vi "Load Named Colors.vi"() -> ()   [LabVIEW 2015, in "ColorSelector.lvclass"]
doc: "This VI is a scripting VI that edits the <b>Named Colors Enum</b> and creates the named colors lookup table from the list in the <b>Named Colors List Text File</b>.\n<b> </b> <b> </b>\n©2017 Q Software Innovations, LLC (QSI)\nwritten by Quentin Alldredge\nproduced in LabVIEW 2015\n\nsupport@qsoftwareinnovations.com\nwww.qsoftwareinnovations.com\n\nAll rights reserved.\n\nRedistribution and use in source and binary forms, with or without modification, are permitted provided that the following conditions are met:\n\n * Redistributions of source code must retain the above copyright notice, this list of conditions and the following disclaimer.\n * Redistributions in binary form must reproduce the above copyright notice, this list of conditions and the following disclaimer in the documentation and/or other materials provided with the distribution.\n * Neither the name of Q Software Innovations, LLC. nor the names of its contributors may be used to endorse or promote products derived from this software without specific prior written permission.\n\nTHIS SOFTWARE IS PROVIDED BY THE COPYRIGHT HOLDERS AND CONTRIBUTORS \"AS IS\" AND ANY EXPRESS OR IMPLIED WARRANTIES, INCLUDING, BUT NOT LIMITED TO, THE IMPLIED WARRANTIES OF MERCHANTABILITY AND FITNESS FOR A PARTICULAR PURPOSE ARE DISCLAIMED. IN NO EVENT SHALL THE COPYRIGHT OWNER OR CONTRIBUTORS BE LIABLE FOR ANY DIRECT, INDIRECT, INCIDENTAL, SPECIAL, EXEMPLARY, OR CONSEQUENTIAL DAMAGES (INCLUDING, BUT NOT LIMITED TO, PROCUREMENT OF SUBSTITUTE GOODS OR SERVICES; LOSS OF USE, DATA, OR PROFITS; OR BUSINESS INTERRUPTION) HOWEVER CAUSED AND ON ANY THEORY OF LIABILITY, WHETHER IN CONTRACT, STRICT LIABILITY, OR TORT (INCLUDING NEGLIGENCE OR OTHERWISE) ARISING IN ANY WAY OUT OF THE USE OF THIS SOFTWARE, EVEN IF ADVISED OF THE POSSIBILITY OF SUCH DAMAGE."
uses:
  ColorSelector.lvclass
  <vilib>/Utility/traverseref.llb/TRef TravTarget.ctl
  <vilib>/Utility/file.llb/Read Delimited Spreadsheet (string).vi
  <vilib>/Utility/traverseref.llb/VI Scripting - Traverse.lvlib
panel:
  out "Lookup Table":variant
  out "sorted array":cluster{"offset past number":u32, string}[](array[cluster])
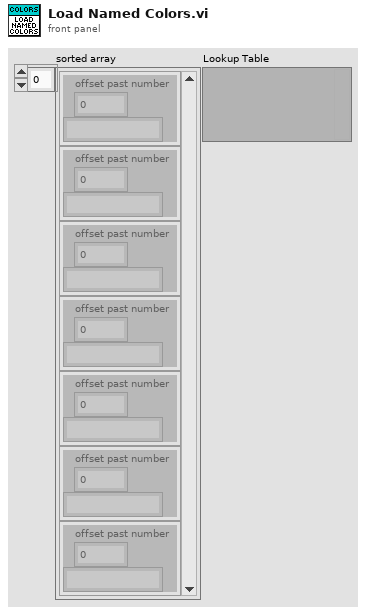
[diagram p1: front panel]
types:
  T1 = typedef "TRef TravTarget.ctl" = enum16{"FP", "BD", "Other"}
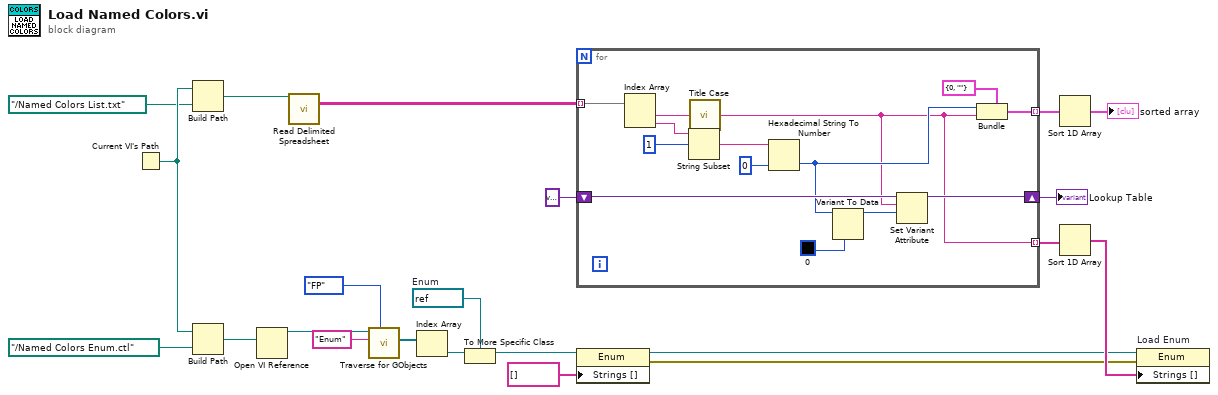
[diagram p0: block diagram]
diagram:
  w13 = refnum<vi> refnum  # Enum
  n1 = Current VI's Path() -> (path=w2:path)
  n2 = Build Path(base path=w2, name or relative path=path "../Named Colors List.txt") -> (appended path=w3:path)
  n3 = Build Path(base path=w2, name or relative path=path "../Named Colors Enum.ctl") -> (appended path=w4:path)
  n4 = Open VI Reference(vi path=w4) -> (vi reference=w18:refnum<vi>)  [unwired: 5 in, 1 out]
  n5 = call-poly <vilib>:"Read Delimited Spreadsheet.vi"("file path (dialog if empty)"=w3) -> ("all rows"=w22:string[][])  [unwired: 9 in, 5 out]
  n6 = call <vilib>:"Traverse for GObjects.vi"("Traverse Target"=TRef_TravTarget."FP", "Class Name"="Enum", "VI Refnum"=w18) -> ("References"=w15:refnum<vi>[])  [unwired: 5 in, 3 out]
  n7 = Index Array(array=w15) -> (element=w14:refnum<vi>)  [unwired: 1 in]
  n8 = To More Specific Class(target class=w13, reference=w14) -> (specific class reference=w8:refnum<vi>)  [unwired: 1 in, 1 out]
  n9 = for {
    tunnel: w22 -> [w36] mode=indexing
    tunnel: [w33] -> w20 mode=indexing
    shift-right: [w32] -> w12
    shift-left: variant -> [w31]
    tunnel: [w24] -> w11 mode=indexing
    n10 = Index Array(array=w36) -> (element #1=w23:string, element #2=w34:string)  [unwired: 2 in]
    n11 = String Subset(string=w34, offset (0)=1) -> (substring=w25:string)  [unwired: 1 in]
    n12 = call "Title Case.vi"("String in"=w23) -> ("String out"=w24:string)
    n13 = Hexadecimal String To Number(string=w25, default (0uL)=u32 0) -> (number=w28:u32)  [unwired: 1 in, 1 out]
    n14 = Variant To Data(type=u32 0, Variant=w28) -> (data=w26:u32)  [unwired: 1 in, 1 out]
    n15 = Set Variant Attribute(Variant=w31, name=w24, value=w26) -> (Variant out=w32:variant)  [unwired: 1 in, 2 out]
    n16 = Bundle(cluster=cluster{"offset past number":u32, string} {"offset past number"=0, ""}, "offset past number"=w28, w24) -> (w33:cluster{"offset past number":u32, string})
  }
  "Lookup Table" <- w12
  n17 = property class="Enum"(reference=w8, "Strings []"=string[] []) -> (reference out=w7:refnum<vi>, error out=w9:errorcluster)  [unwired: 1 in]
  n18 = Sort 1D Array(array=w20) -> (sorted array=→"sorted array":cluster{"offset past number":u32, string}[])
  n19 = Sort 1D Array(array=w11) -> (sorted array=w10:string[])
  n20 = property on="Load Enum" class="Enum"(reference=w7, error in=w9, "Strings []"=w10) -> ()  [unwired: 2 out]
